vi "SeCrTs-Edit Channel Name list.vi"() -> ()   [LabVIEW 2022 SP3]
uses:
  Controls/SeCrTs-Edit CHN names.ctl
panel:
  out "Signal names":string[][](array[string])
  in  "Exit":bool
  in  "Save":bool
  in  "Select file to Edit":path
  out "List":string[](array[string])
  in  "Listbox":i32(listbox)
  in  "Tab Control":enum32{"Add New Name", "Rename"}(tab)
  in  "Add to list":bool
  in  "Channel Name":string[](array[string])
  in  "Enter New Name":string
  in  "Choose Channel names":string(combo)
  in  "Rename":bool
  in  "Delete":bool
  # "Channel Name Editor"
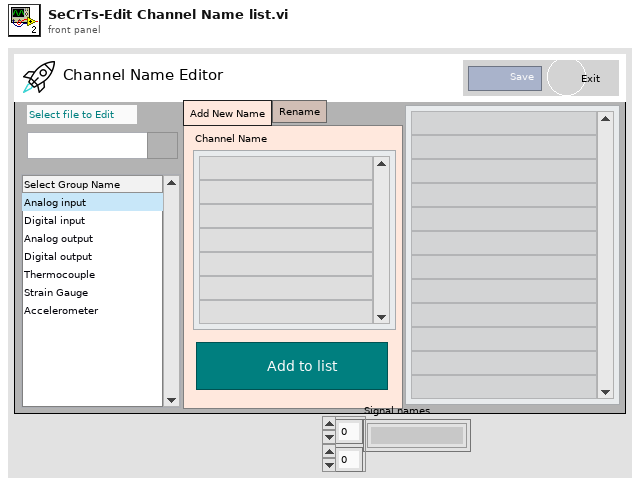
[diagram p1: front panel]
types:
  T1 = typedef "SeCrTs-Edit CHN names.ctl" = enum16{"initialize", "select group", "rename", "add to list", "pollevent", "Quit", "Save", "Read"}
  T2 = cluster{"path":path, "Data":string[][], "Group":i32}
  T3 = enum16{"open", "replace", "create", "open or create", "replace or create", "replace or create with confirmation"}
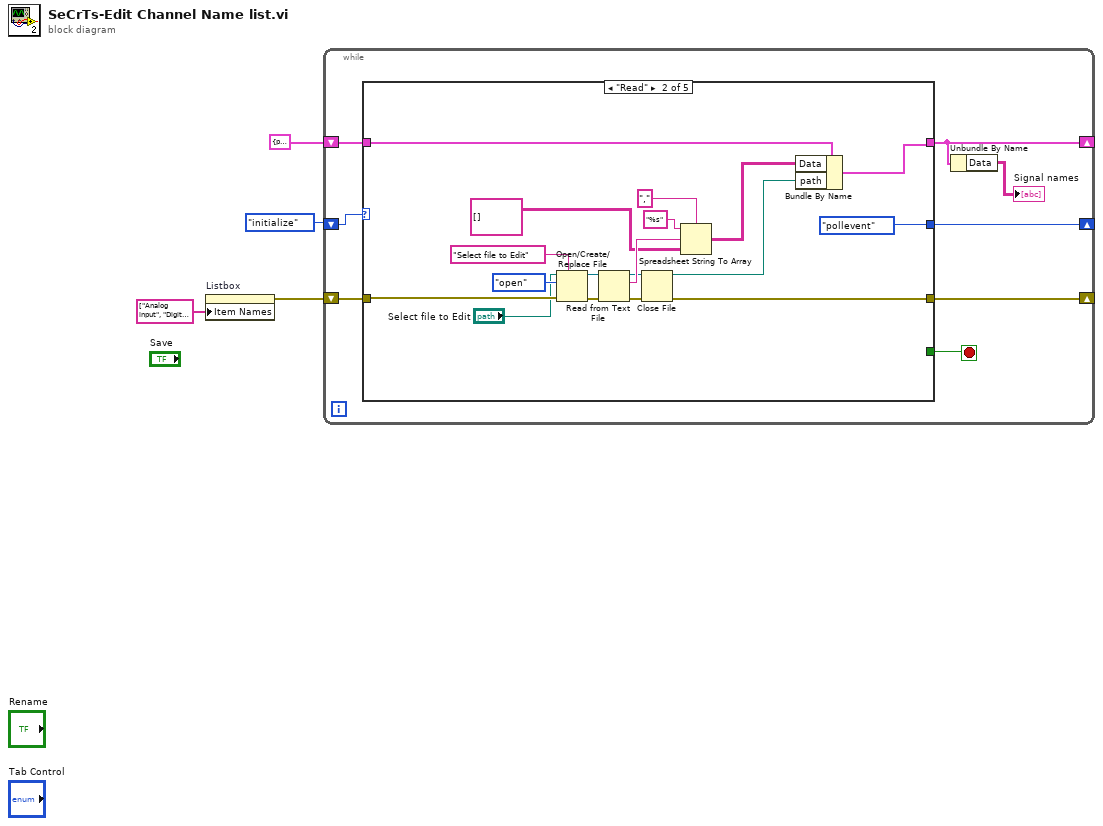
[diagram p0: block diagram]
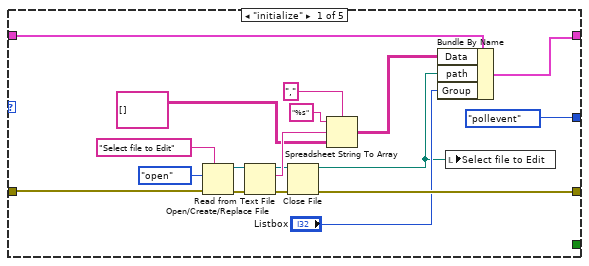
[diagram p2: hidden frame]
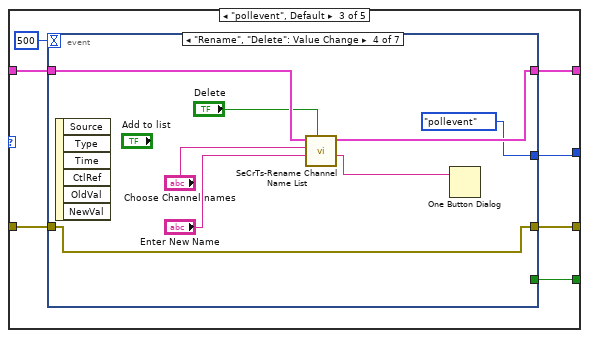
[diagram p3: hidden frame]
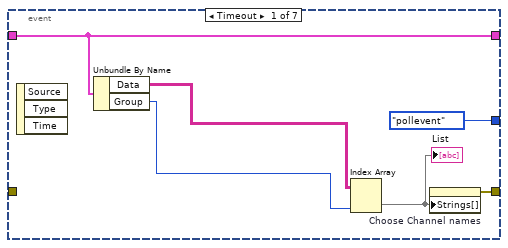
[diagram p4: hidden frame]
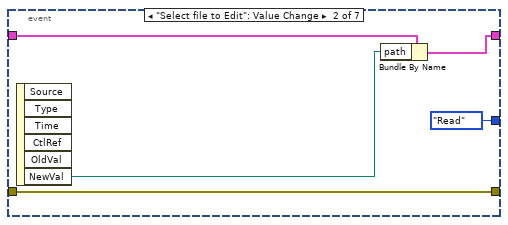
[diagram p5: hidden frame]
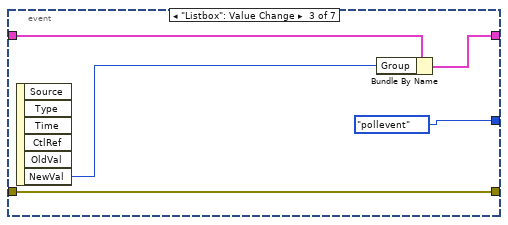
[diagram p6: hidden frame]
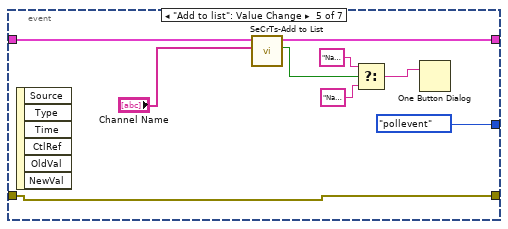
[diagram p7: hidden frame]
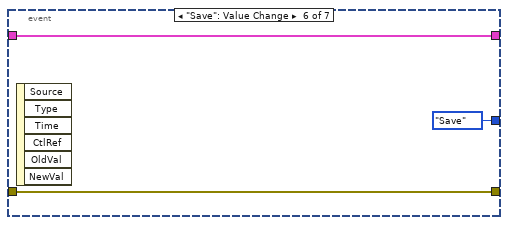
[diagram p8: hidden frame]
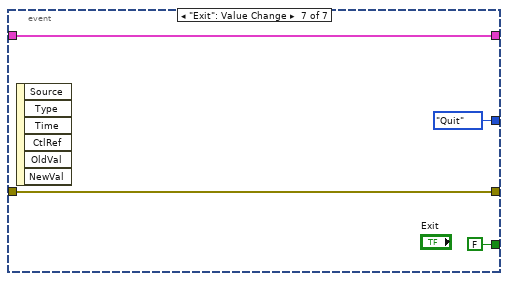
[diagram p9: hidden frame]
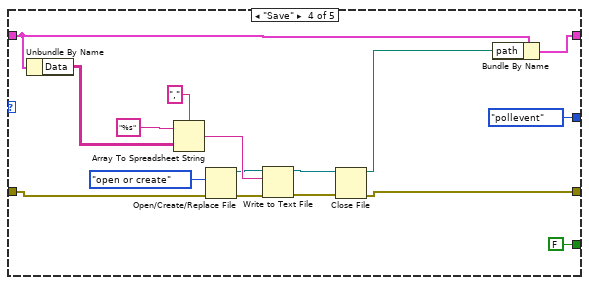
[diagram p10: hidden frame]
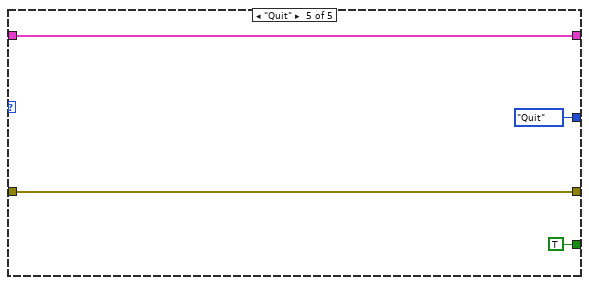
[diagram p11: hidden frame]
diagram:
  n1 = property on="Listbox" class="LstBox (strict)"("Item Names"=string[] ["Analog input", "Digital input", "Analog output", "Digital output", "Thermocouple", "Strain Gauge", "Accelerometer"]) -> (error out=w3:errorcluster)  [unwired: 2 in, 1 out]
  n2 = while {
    shift-right: [w6] -> _
    shift-left: T2 {"path"=path "", "Data"=[], "Group"=0} -> [w11]
    shift-right: [w9] -> _
    shift-left: w3 -> [w10]
    shift-right: [w8] -> _
    shift-left: SeCrTs-Edit_CHN_names."initialize" -> [w12]
    stop <- w7 stop-if-true
    n3 = case shown="\"Read\"" w12 {
      tunnel: w11 -> [w18 w36 w55 w100 w112]
      tunnel: [w16 w34 w54 w103 w112] -> w6
      tunnel: w10 -> [w20 w38 w51 w104 w113]
      tunnel: [w19 w37 w52 w105 w113] -> w9
      tunnel: [SeCrTs-Edit_CHN_names."pollevent" SeCrTs-Edit_CHN_names."pollevent" w53 SeCrTs-Edit_CHN_names."pollevent" SeCrTs-Edit_CHN_names."Quit"] -> w8
      tunnel: [_ _ w49 FALSE ("Quit") TRUE ("Quit")] -> w7
      frame "initialize" {
        n4 = Open/Create/Replace File(error in=w20, prompt="Select file to Edit", operation (0:open)=T3."open") -> (refnum out=w27:refnum<file>, error out=w26:errorcluster)  [unwired: 3 in, 1 out]
        n5 = Read from Text File(file (use dialog)=w27, error in=w26) -> (refnum out=w29:refnum<file>, text=w30:string, error out=w28:errorcluster)  [unwired: 2 in, 1 out]
        n6 = Close File(refnum=w29, error in=w28) -> (path=w13:path, error out=w19:errorcluster)
        n7 = Spreadsheet String To Array(delimiter (Tab)=",", format string="%s", spreadsheet string=w30, array type (2D Dbl)=string[][] [] ("Table Control")) -> (array=w17:string[][])
        n8 = Bundle By Name(cluster=w18, "Data"=w17, "path"=w13, "Group"="Listbox") -> (w16:T2)
        n9 = local write "Select file to Edit"(w13) -> ()
      }
      frame "Read" {
        n10 = Open/Create/Replace File(file path (use dialog)="Select file to Edit", error in=w38, prompt="Select file to Edit", operation (0:open)=T3."open") -> (refnum out=w45:refnum<file>, error out=w44:errorcluster)  [unwired: 2 in, 1 out]
        n11 = Read from Text File(file (use dialog)=w45, error in=w44) -> (refnum out=w47:refnum<file>, text=w48:string, error out=w46:errorcluster)  [unwired: 2 in, 1 out]
        n12 = Close File(refnum=w47, error in=w46) -> (path=w33:path, error out=w37:errorcluster)
        n13 = Spreadsheet String To Array(delimiter (Tab)=",", format string="%s", spreadsheet string=w48, array type (2D Dbl)=string[][] [] ("Table Control")) -> (array=w35:string[][])
        n14 = Bundle By Name(cluster=w36, "Data"=w35, "path"=w33) -> (w34:T2)
      }
      frame "pollevent", Default {
        n15 = event shown="[3] \"Rename\", \"Delete\": Value Change" {
          selector: _ -> [_ _ _ _ _ _ _]
          dyn-events: _ -> [_ _ _ _ _ _ _]
          timeout: 500 -> [_ _ _ _ _ _ _]
          tunnel: w55 -> [w60 w65 w70 w78 w87 w91 w94]
          tunnel: [w60 w66 w71 w79 w88 w91 w94] -> w54
          tunnel: [SeCrTs-Edit_CHN_names."pollevent" SeCrTs-Edit_CHN_names."Read" SeCrTs-Edit_CHN_names."pollevent" SeCrTs-Edit_CHN_names."pollevent" SeCrTs-Edit_CHN_names."pollevent" SeCrTs-Edit_CHN_names."Save" SeCrTs-Edit_CHN_names."Quit"] -> w53
          tunnel: [w61 w62 w68 w75 w81 w89 w92] -> w52
          tunnel: w51 -> [_ w62 w68 w75 w81 w89 w92]
          tunnel: [_ _ _ _ _ _ FALSE ("Quit")] -> w49
          event Timeout {
            n16 = event-data() -> ()  [unwired: 1 in, 3 out]
            n17 = Unbundle By Name(w60) -> ("Data"=w59:string[][], "Group"=w57:i32)
            n18 = Index Array(array=w59, index (col)=w57) -> (element=w58:string[])  [unwired: 1 in]
            "List" <- w58
            n19 = property on="Choose Channel names" class="CmbBox"("Strings[]"=w58) -> (error out=w61:errorcluster)  [unwired: 2 in, 1 out]
          }
          event "Select file to Edit": Value Change {
            n20 = event-data() -> ("NewVal"=w64:path)  [unwired: 1 in, 5 out]
            n21 = Bundle By Name(cluster=w65, "path"=w64) -> (w66:T2)
          }
          event "Listbox": Value Change {
            n22 = event-data() -> ("NewVal"=w69:i32)  [unwired: 1 in, 5 out]
            n23 = Bundle By Name(cluster=w70, "Group"=w69) -> (w71:T2)
          }
          event "Rename", "Delete": Value Change {
            n24 = event-data() -> ()  [unwired: 1 in, 6 out]
            n25 = call "SeCrTs-Rename Channel Name List.vi"("delete (T)"="Delete", "Enter New Name"="Enter New Name", "Choose Channel names"="Choose Channel names", "Cluster in"=w78) -> ("dialog"=w72:string, "Cluster out"=w79:T2)  [unwired: 6 in]
            n26 = One Button Dialog(message=w72) -> ()  [unwired: 1 in, 1 out]
          }
          event "Add to list": Value Change {
            n27 = event-data() -> ()  [unwired: 1 in, 6 out]
            n28 = call "SeCrTs-Add to List.vi"("Enter Channel Name"="Channel Name", "Cluster in"=w87) -> ("Boolean"=w83:bool, "Cluster out"=w88:T2)  [unwired: 8 in]
            n29 = Select(t="Name You Entered is already Exist!" ("message"), s=w83, f="Name Successfully Changed.") -> (s? t:f=w85:string)
            n30 = One Button Dialog(message=w85) -> ()  [unwired: 1 in, 1 out]
          }
          event "Save": Value Change {
            n31 = event-data() -> ()  [unwired: 1 in, 6 out]
          }
          event "Exit": Value Change {
            n32 = event-data() -> ()  [unwired: 1 in, 6 out]
          }
        }
      }
      frame "Save" {
        n33 = Unbundle By Name(w100) -> ("Data"=w96:string[][])
        n34 = Array To Spreadsheet String(delimiter (Tab)=",", array=w96, 3:"%s" ("format string")) -> (spreadsheet string=w111:string)
        n35 = Open/Create/Replace File(error in=w104, operation (0:open)=T3."open or create") -> (refnum out=w110:refnum<file>, error out=w99:errorcluster)  [unwired: 4 in, 1 out]
        n36 = Write to Text File(file (use dialog)=w110, text=w111, error in=w99) -> (refnum out=w109:refnum<file>, error out=w98:errorcluster)  [unwired: 1 in, 1 out]
        n37 = Close File(refnum=w109, error in=w98) -> (path=w101:path, error out=w105:errorcluster)
        n38 = Bundle By Name(cluster=w100, "path"=w101) -> (w103:T2)
      }
      frame "Quit" {
      }
    }
    n39 = Unbundle By Name(w6) -> ("Data"=→"Signal names":string[][])
  }
